vi "Activate Feature.vi"(6 "Remote Timeout (300,000 ms)":u32=300000, 8 "error in (no error)":errorcluster, 9 "Activation Code":string, 10 "Feature ID":u32 format="%0x", 11 "Resource in":refnum<k20>) -> (0 "error out":errorcluster, 2 "Detailed Result":string, 3 "Resource out":refnum<k20>)   [LabVIEW 2020, in "nisyscfg.lvlib"]
doc: "Activates a feature of the hardware using an activation code provided by NI."
uses:
  <vilib>/nisyscfg/nisyscfg.lvlib
  <vilib>/Utility/error.llb/Error Cluster From Error Code.vi
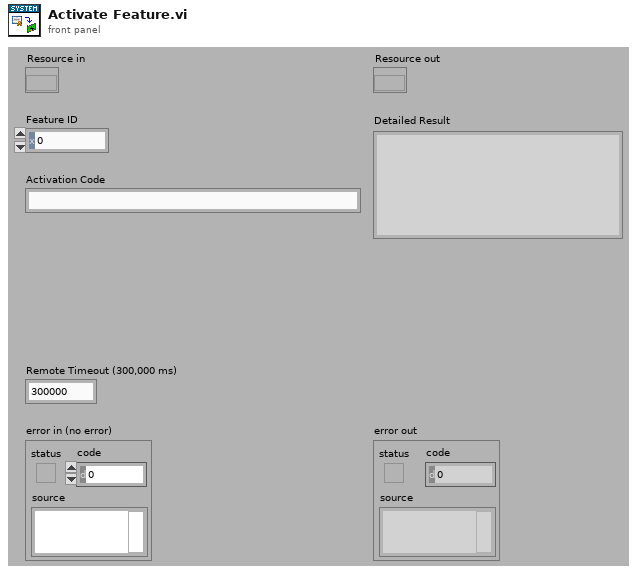
[diagram p1: front panel]
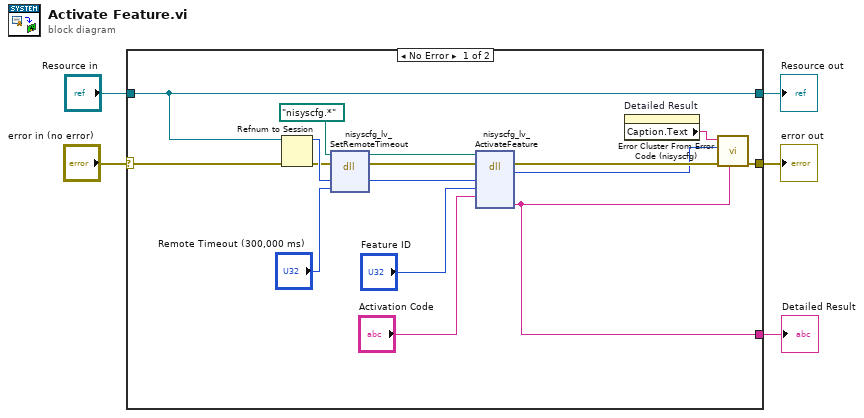
[diagram p0: block diagram]
diagram:
  n1 = case shown="No Error" "error in (no error)" {
    selector: "error in (no error)" -> [w11 w23]
    tunnel: [w21 w23] -> w5
    tunnel: "Resource in" -> [w10 w22]
    tunnel: [w8 _] -> w1
    tunnel: [w10 w22] -> w2
    frame No Error {
      n2 = Refnum to Session(4:w11, 7:w10) -> (0:w17:errorcluster, 3:w18:u64)
      n3 = dll-call lib="nisyscfg.*" fn="nisyscfg_lv_SetRemoteTimeout" label="SetRemoteTimeout"(path in=path "nisyscfg.*", error in=w17, "item"=w18, "connectTimeout"="Remote Timeout (300,000 ms)") -> (path out=w12:path, error out=w14:errorcluster, "item"=w13:u64)  [unwired: 1 in, 2 out]
      n4 = dll-call lib="nisyscfg.*" fn="nisyscfg_lv_ActivateFeature" label="ActivateFeature"(path in=w12, error in=w14, "itemHandle"=w13, "featureID"="Feature ID", "activationCode"="Activation Code") -> (error out=w20:errorcluster, "return type"=w19:i32, "details"=w8:string)  [unwired: 5 in, 1 out]
      n5 = property on="Detailed Result" class="Str"() -> ("Caption.Text"=w9:string)  [unwired: 2 in, 2 out]
      n6 = call <vilib>:"Error Cluster From Error Code (nisyscfg).vi"("Details String"=w8, "error in (no error)"=w20, "Error Code (0)"=w19, "Details Caption"=w9) -> ("error out"=w21:errorcluster)  [unwired: 7 in]
    }
    frame Error {
    }
  }
  "error out" <- w5
  "Resource out" <- w2
  "Detailed Result" <- w1
